vi "Initialize Tree with Plugins.vi"(8 "error in (no error)":errorcluster, 11 "Application Data in":T1) -> (0 "error out":errorcluster, 3 "Application Data out":T1)   [LabVIEW 2017, in "DSF Data Viewer.lvlib"]
uses:
  DSF Data Viewer.lvlib
  Application Data.ctl
  Core/Engine/Classes/Framework/Framework.lvclass
  View Mode.ctl
  Core/Engine/Classes/Framework/Framework.lvclass/Framework.ctl
  Core/Engine/Classes/Plugin/Plugin.lvclass/Plugin.ctl
  Item Tree/ID to Tree Items/Plugin ID to Tree Items.vi
  Core/Engine/Classes/Framework/Get Async Plugins.vi
  Core/Engine/Classes/Framework/Get Inline Plugins.vi
  Item Tree/Create New Tree Item.vi
  Core/Engine/Classes/Plugin/Get Name.vi
  Item Tree/Add Item to Tree.vi
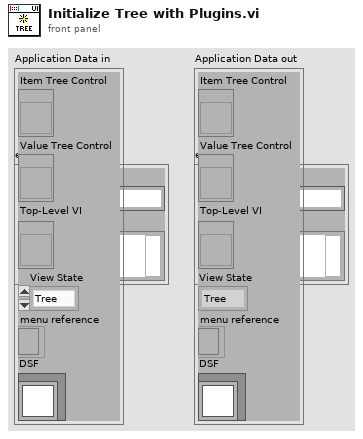
[diagram p1: front panel]
types:
  T1 = typedef "DSF Data Viewer.lvlib/Application Data.ctl" = cluster{"Item Tree Control":refnum<vi>, "Value Tree Control":refnum<vi>, "Top-Level VI":refnum<vi>, "View State":T2, "menu reference":refnum<k9>, "DSF":refnum<class "Framework.lvclass">}
  T2 = typedef "DSF Data Viewer.lvlib/View Mode.ctl" = enum16{"Tree", "List"}
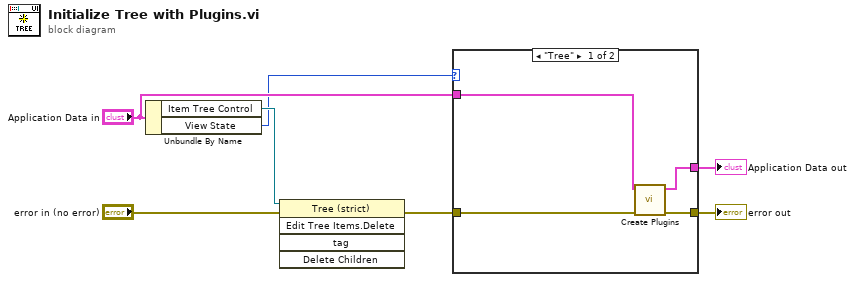
[diagram p0: block diagram]
diagram:
  n1 = Unbundle By Name("Application Data in") -> ("Item Tree Control"=w2:refnum<vi>, "View State"=w1:T2)
  n2 = invoke class="Tree (strict)" method="Edit Tree Items.Delete"(reference=w2, error in="error in (no error)") -> (error out=w5:errorcluster)  [unwired: 3 in, 4 out]
  n3 = case shown="\"Tree\"" w1 {
    tunnel: "Application Data in" -> [w8 w13]
    tunnel: w5 -> [w11 w12]
    tunnel: [w9 w12] -> w4
    tunnel: [w10 w13] -> w3
    frame "Tree" {
      n4 = call "Create Plugins.vi"("error in (no error)"=w11, "Application Data In"=w8) -> ("error out"=w9:errorcluster, "Application Data out"=w10:T1)  [unwired: 8 in]
    }
    frame "List" {
    }
  }
  "error out" <- w4
  "Application Data out" <- w3
